vi "HandleObservationSync.vi"(8 "error in (no error)":errorcluster, 11 "S4GUI in":refnum<class "S4GUI.lvclass">) -> (0 "error out":errorcluster, 3 "S4GUI out":refnum<class "S4GUI.lvclass">)   [LabVIEW 2018, in "S4GUI.lvclass"] (continued)
              n1024 = call-dynamic "Read Channel.vi"("error in (no error)"=w2761, "Acquisition in"=w2762) -> ("error out"=w2769:errorcluster, "Channel.lvclass"=w2770:refnum<class "Channel.lvclass">, "Acquisition out"=w2763:refnum<class "Acquisition.lvclass">)  [unwired: 7 in]
              n1025 = call-dynamic "Read State Machine.vi"("error in (no error)"=w2769, "Device in"=w2770) -> ("error out"=w2768:errorcluster, "State Machine.lvclass"=w2766:refnum<class "State Machine.lvclass">, "Device out"=w2772:refnum<class "Channel.lvclass">)  [unwired: 7 in]
              n1026 = call "Next State.vi"("error in (no error)"=w2768, "New_State"=50, "State Machine in"=w2766) -> ("error out"=w2760:errorcluster, "State Machine out"=w2759:refnum<class "State Machine.lvclass">)  [unwired: 7 in]
              n1027 = call-dynamic "Write State Machine.vi"("error in (no error)"=w2760, "State Machine.lvclass"=w2759, "Device in"=w2772) -> ("error out"=w2773:errorcluster, "Device out"=w2771:refnum<class "Channel.lvclass">)  [unwired: 7 in]
              n1028 = call-dynamic "Write Channel.vi"("error in (no error)"=w2773, "Channel.lvclass"=w2771, "Acquisition in"=w2763) -> ("error out"=w2765:errorcluster, "Acquisition out"=w2764:refnum<class "Acquisition.lvclass">)  [unwired: 7 in]
            }
          }
          n1029 = call-dynamic "Write AcquisitionC.vi"("error in (no error)"=w2684, "Acquisition.lvclass"=w2682, "S4ACS_GUI in"=w2683) -> ("error out"=w2678:errorcluster, "S4ACS_GUI out"=w2677:refnum<class "S4GUI.lvclass">)  [unwired: 7 in]
          n1030 = call-dynamic "Read AcquisitionD.vi"("error in (no error)"=w2678, "S4ACS_GUI in"=w2677) -> ("error out"=w2634:errorcluster, "Acquisition.lvclass"=w2636:refnum<class "Acquisition.lvclass">, "S4ACS_GUI out"=w2676:refnum<class "S4GUI.lvclass">)  [unwired: 7 in]
          n1031 = call-dynamic "Read enabled.vi"("error in (no error)"=w2634, "Server in"=w2636) -> ("error out"=w2633:errorcluster, "enabled"=w2629:bool, "Server out"=w2635:refnum<class "Acquisition.lvclass">)  [unwired: 7 in]
          n1032 = call "Read connection.vi"("error in (no error)"=w2633, "Server in"=w2635) -> ("error out"=w2665:errorcluster, "connection"=w2649:bool, "Server out"=w2666:refnum<class "Acquisition.lvclass">)  [unwired: 7 in]
          n1033 = And(x=w2649, y=w2629) -> (x .and. y?=w2651:bool)
          n1034 = case shown="True" w2651 {
            tunnel: w2665 -> [w2734 w2751]
            tunnel: [w2734 w2750] -> w2679
            tunnel: w2666 -> [w2735 w2741]
            tunnel: [w2735 w2739] -> w2675
            tunnel: [w2731 u32 0 ("New_State")] -> w2658
            tunnel: w2629 -> [w2730 _]
            frame False {
              n1035 = Select(t=u32 8, s=w2730, f=u32 0) -> (s? t:f=w2731:u32)
            }
            frame True {
              n1036 = call-dynamic "Read Channel.vi"("error in (no error)"=w2751, "Acquisition in"=w2741) -> ("error out"=w2746:errorcluster, "Channel.lvclass"=w2745:refnum<class "Channel.lvclass">, "Acquisition out"=w2740:refnum<class "Acquisition.lvclass">)  [unwired: 7 in]
              n1037 = call-dynamic "Read State Machine.vi"("error in (no error)"=w2746, "Device in"=w2745) -> ("error out"=w2747:errorcluster, "State Machine.lvclass"=w2749:refnum<class "State Machine.lvclass">, "Device out"=w2743:refnum<class "Channel.lvclass">)  [unwired: 7 in]
              n1038 = call "Next State.vi"("error in (no error)"=w2747, "New_State"=50, "State Machine in"=w2749) -> ("error out"=w2737:errorcluster, "State Machine out"=w2738:refnum<class "State Machine.lvclass">)  [unwired: 7 in]
              n1039 = call-dynamic "Write State Machine.vi"("error in (no error)"=w2737, "State Machine.lvclass"=w2738, "Device in"=w2743) -> ("error out"=w2742:errorcluster, "Device out"=w2744:refnum<class "Channel.lvclass">)  [unwired: 7 in]
              n1040 = call-dynamic "Write Channel.vi"("error in (no error)"=w2742, "Channel.lvclass"=w2744, "Acquisition in"=w2740) -> ("error out"=w2750:errorcluster, "Acquisition out"=w2739:refnum<class "Acquisition.lvclass">)  [unwired: 7 in]
            }
          }
          n1041 = call-dynamic "Write AcquisitionD.vi"("error in (no error)"=w2679, "Acquisition.lvclass"=w2675, "S4ACS_GUI in"=w2676) -> ("error out"=w2674:errorcluster, "S4ACS_GUI out"=w2673:refnum<class "S4GUI.lvclass">)  [unwired: 7 in]
          n1042 = Compound Arithmetic op=ADD(w2661, w2660, w2659, w2658) -> (w2662:u32)
          n1043 = case shown="0, Default" w2662 {
            tunnel: w2657 -> [w2699 _ _ _ _ _ _ _ _ _ _ _ _ _ _ _]
            tunnel: [w2698 u32 1 ("Obs_state") u32 1 ("Obs_state") u32 1 ("Obs_state") u32 1 ("Obs_state") u32 1 ("Obs_state") u32 1 ("Obs_state") u32 1 ("Obs_state") u32 1 ("Obs_state") u32 1 ("Obs_state") u32 1 ("Obs_state") u32 1 ("Obs_state") u32 1 ("Obs_state") u32 1 ("Obs_state") u32 1 ("Obs_state") u32 1 ("Obs_state")] -> w2663
            tunnel: ["" ("Error Msg") "ERROR: Lost channel 1 connection... - HandleObservationSync.vi state 308" ("Error Msg") "ERROR: Lost channel 2 connection...- HandleObservationSync.vi state 308" ("Error Msg") "ERROR: Lost channels 1 and 2 connection...- HandleObservationSync.vi state 308" ("Error Msg") "ERROR: Lost channel 3 connection...- HandleObservationSync.vi state 308" ("Error Msg") "ERROR: Lost channels 1 and  3 connection...- HandleObservationSync.vi state 308" ("Error Msg") "ERROR:  Lost channels 2 and  3 connection...- HandleObservationSync.vi state 308" ("Error Msg") "ERROR:  Lost channels 1, 2 and  3 connection...- HandleObservationSync.vi state 308" ("Error Msg") "ERROR: Lost channel 4 connection...- HandleObservationSync.vi state 308" ("Error Msg") "ERROR:  Lost channels 1 and 4 connection...- HandleObservationSync.vi state 308" ("Error Msg") "ERROR:  Lost channels 2 and 4 connection...- HandleObservationSync.vi state 308" ("Error Msg") "ERROR: Lost channels 1, 2 and 4 connection...- HandleObservationSync.vi state 308" ("Error Msg") "ERROR: Lost channels 3 and 4 connection...- HandleObservationSync.vi state 308" ("Error Msg") "ERROR: Lost channels 1, 3 and 4 connection...- HandleObservationSync.vi state 308" ("Error Msg") "ERROR: Lost channels 2, 3 and 4 connection...- HandleObservationSync.vi state 308" ("Error Msg") "ERROR: Lost channels 1, 2, 3 and 4 connection...- HandleObservationSync.vi state 308" ("Error Msg")] -> w2664
            frame 0, Default {
              n1044 = Tick Count (ms)() -> (millisecond timer value=w2696:u32)
              n1045 = Increment(x=w2699) -> (x+1=w2698:u32)
              n1046 = local write "time1"(w2696) -> ()
            }
            frame 1 {
            }
            frame 2 {
            }
            frame 3 {
            }
            frame 4 {
            }
            frame 5 {
            }
            frame 6 {
            }
            frame 7 {
            }
            frame 8 {
            }
            frame 9 {
            }
            frame 10 {
            }
            frame 11 {
            }
            frame 12 {
            }
            frame 13 {
            }
            frame 14 {
            }
            frame 15 {
            }
          }
          n1047 = Bundle By Name(cluster=w2673, "Obs_state"=w2663, "Error Msg"=w2664) -> (w2690:refnum<class "S4GUI.lvclass">)
        }
        frame 309 {
          # "Se wait_expose=T, não envia\no EXPOSE do estado 310\n(1o EXPOSE já foi enviado).\n\nNeste caso, vai para:\n* 310 se houver mais \n   de 1 posição da lamina ou para \n* 327 se houver apenas 1 posição\n   da lâmina"
          # "T: mode EXPOSE\nF: mode FIRE"
          n1048 = Unbundle By Name(w2824) -> ("seqAtual"=w2823:u32)
          n1049 = call-dynamic "Read AcquisitionA.vi"("error in (no error)"=w2884, "S4ACS_GUI in"=w2824) -> ("error out"=w2864:errorcluster, "Acquisition.lvclass"=w2865:refnum<class "Acquisition.lvclass">, "S4ACS_GUI out"=w2886:refnum<class "S4GUI.lvclass">)  [unwired: 7 in]
          n1050 = call "Read connection.vi"("error in (no error)"=w2864, "Server in"=w2865) -> ("error out"=w2866:errorcluster, "connection"=w2868:bool, "Server out"=w2867:refnum<class "Acquisition.lvclass">)  [unwired: 7 in]
          n1051 = case shown="True" w2868 {
            tunnel: [w3037 w3061] -> w2887
            tunnel: [w3036 w3060] -> w2885
            tunnel: w2867 -> [w3037 w3053]
            tunnel: w2866 -> [w3036 w3052]
            tunnel: [TRUE w3051] -> w2847
            tunnel: [FALSE w3045] -> w2843
            tunnel: [TRUE w3039] -> w2828
            tunnel: w2823 -> [_ w3038]
            frame False {
            }
            frame True {
              n1052 = call-dynamic "Read Channel.vi"("error in (no error)"=w3052, "Acquisition in"=w3053) -> ("error out"=w3042:errorcluster, "Channel.lvclass"=w3044:refnum<class "Channel.lvclass">, "Acquisition out"=w3062:refnum<class "Acquisition.lvclass">)  [unwired: 7 in]
              n1053 = call-dynamic "Read SequesDone.vi"("error in (no error)"=w3042, "Channel in"=w3044) -> ("error out"=w3041:errorcluster, "SequesDoneRaw"=w3040:u32, "Channel out"=w3043:refnum<class "Channel.lvclass">)  [unwired: 6 in, 1 out]
              n1054 = Equal?(x=w3040, y=w3038) -> (x = y?=w3039:bool)
              n1055 = call-dynamic "Read wait_expose.vi"("error in (no error)"=w3041, "Channel in"=w3043) -> ("error out"=w3046:errorcluster, "wait_expose"=w3045:bool, "Channel out"=w3047:refnum<class "Channel.lvclass">)  [unwired: 7 in]
              n1056 = call-dynamic "Read State Machine.vi"("error in (no error)"=w3046, "Device in"=w3047) -> ("error out"=w3054:errorcluster, "State Machine.lvclass"=w3056:refnum<class "State Machine.lvclass">, "Device out"=w3058:refnum<class "Channel.lvclass">)  [unwired: 7 in]
              n1057 = call-dynamic "Read State.vi"("error in (no error)"=w3054, "State Machine in"=w3056) -> ("error out"=w3048:errorcluster, "State"=w3050:i32, "State Machine out"=w3055:refnum<class "State Machine.lvclass">)  [unwired: 7 in]
              n1058 = Greater?(x=w3050, y=53) -> (0:w3051:bool)
              n1059 = call-dynamic "Write State Machine.vi"("error in (no error)"=w3048, "State Machine.lvclass"=w3055, "Device in"=w3058) -> ("error out"=w3057:errorcluster, "Device out"=w3059:refnum<class "Channel.lvclass">)  [unwired: 7 in]
              n1060 = call-dynamic "Write Channel.vi"("error in (no error)"=w3057, "Channel.lvclass"=w3059, "Acquisition in"=w3062) -> ("error out"=w3060:errorcluster, "Acquisition out"=w3061:refnum<class "Acquisition.lvclass">)  [unwired: 7 in]
            }
          }
          n1061 = call-dynamic "Write AcquisitionA.vi"("error in (no error)"=w2885, "Acquisition.lvclass"=w2887, "S4ACS_GUI in"=w2886) -> ("error out"=w2881:errorcluster, "S4ACS_GUI out"=w2882:refnum<class "S4GUI.lvclass">)  [unwired: 7 in]
          n1062 = call "Read AcquisitionB.vi"("error in (no error)"=w2881, "S4ACS_GUI in"=w2882) -> ("error out"=w2861:errorcluster, "Acquisition.lvclass"=w2863:refnum<class "Acquisition.lvclass">, "S4ACS_GUI out"=w2879:refnum<class "S4GUI.lvclass">)  [unwired: 7 in]
          n1063 = call "Read connection.vi"("error in (no error)"=w2861, "Server in"=w2863) -> ("error out"=w2860:errorcluster, "connection"=w2859:bool, "Server out"=w2862:refnum<class "Acquisition.lvclass">)  [unwired: 7 in]
          n1064 = case shown="True" w2859 {
            tunnel: w2862 -> [w3007 w3032]
            tunnel: w2860 -> [w3006 w3031]
            tunnel: [w3007 w3029] -> w2880
            tunnel: [w3006 w3028] -> w2878
            tunnel: [TRUE w3019] -> w2846
            tunnel: [FALSE ("expose") w3015] -> w2842
            tunnel: [TRUE w3009] -> w2830
            tunnel: w2823 -> [_ w3008]
            frame False {
            }
            frame True {
              n1065 = call-dynamic "Read Channel.vi"("error in (no error)"=w3031, "Acquisition in"=w3032) -> ("error out"=w3011:errorcluster, "Channel.lvclass"=w3014:refnum<class "Channel.lvclass">, "Acquisition out"=w3030:refnum<class "Acquisition.lvclass">)  [unwired: 7 in]
              n1066 = call-dynamic "Read SequesDone.vi"("error in (no error)"=w3011, "Channel in"=w3014) -> ("error out"=w3010:errorcluster, "SequesDoneRaw"=w3012:u32, "Channel out"=w3013:refnum<class "Channel.lvclass">)  [unwired: 6 in, 1 out]
              n1067 = Equal?(x=w3012, y=w3008) -> (x = y?=w3009:bool)
              n1068 = call-dynamic "Read wait_expose.vi"("error in (no error)"=w3010, "Channel in"=w3013) -> ("error out"=w3016:errorcluster, "wait_expose"=w3015:bool, "Channel out"=w3017:refnum<class "Channel.lvclass">)  [unwired: 7 in]
              n1069 = call-dynamic "Read State Machine.vi"("error in (no error)"=w3016, "Device in"=w3017) -> ("error out"=w3022:errorcluster, "State Machine.lvclass"=w3024:refnum<class "State Machine.lvclass">, "Device out"=w3026:refnum<class "Channel.lvclass">)  [unwired: 7 in]
              n1070 = call-dynamic "Read State.vi"("error in (no error)"=w3022, "State Machine in"=w3024) -> ("error out"=w3021:errorcluster, "State"=w3018:i32, "State Machine out"=w3023:refnum<class "State Machine.lvclass">)  [unwired: 7 in]
              n1071 = Greater?(x=w3018, y=53) -> (0:w3019:bool)
              n1072 = call-dynamic "Write State Machine.vi"("error in (no error)"=w3021, "State Machine.lvclass"=w3023, "Device in"=w3026) -> ("error out"=w3025:errorcluster, "Device out"=w3027:refnum<class "Channel.lvclass">)  [unwired: 7 in]
              n1073 = call-dynamic "Write Channel.vi"("error in (no error)"=w3025, "Channel.lvclass"=w3027, "Acquisition in"=w3030) -> ("error out"=w3028:errorcluster, "Acquisition out"=w3029:refnum<class "Acquisition.lvclass">)  [unwired: 7 in]
            }
          }
          n1074 = call "Write AcquisitionB.vi"("error in (no error)"=w2878, "Acquisition.lvclass"=w2880, "S4ACS_GUI in"=w2879) -> ("error out"=w2874:errorcluster, "S4ACS_GUI out"=w2873:refnum<class "S4GUI.lvclass">)  [unwired: 7 in]
          n1075 = call-dynamic "Read AcquisitionC.vi"("error in (no error)"=w2874, "S4ACS_GUI in"=w2873) -> ("error out"=w2856:errorcluster, "Acquisition.lvclass"=w2858:refnum<class "Acquisition.lvclass">, "S4ACS_GUI out"=w2876:refnum<class "S4GUI.lvclass">)  [unwired: 7 in]
          n1076 = call "Read connection.vi"("error in (no error)"=w2856, "Server in"=w2858) -> ("error out"=w2855:errorcluster, "connection"=w2854:bool, "Server out"=w2857:refnum<class "Acquisition.lvclass">)  [unwired: 7 in]
          n1077 = case shown="True" w2854 {
            tunnel: [w2976 w2997] -> w2877
            tunnel: [w2977 w2996] -> w2875
            tunnel: w2857 -> [w2977 w2992]
            tunnel: w2855 -> [w2976 w2991]
            tunnel: [TRUE w2988] -> w2845
            tunnel: [FALSE ("expose") w2985] -> w2841
            tunnel: [TRUE w2979] -> w2829
            tunnel: w2823 -> [_ w2978]
            frame False {
            }
            frame True {
              n1078 = call-dynamic "Read Channel.vi"("error in (no error)"=w2991, "Acquisition in"=w2992) -> ("error out"=w2984:errorcluster, "Channel.lvclass"=w2983:refnum<class "Channel.lvclass">, "Acquisition out"=w2995:refnum<class "Acquisition.lvclass">)  [unwired: 7 in]
              n1079 = call-dynamic "Read SequesDone.vi"("error in (no error)"=w2984, "Channel in"=w2983) -> ("error out"=w2980:errorcluster, "SequesDoneRaw"=w2981:u32, "Channel out"=w2982:refnum<class "Channel.lvclass">)  [unwired: 6 in, 1 out]
              n1080 = Equal?(x=w2981, y=w2978) -> (x = y?=w2979:bool)
              n1081 = call-dynamic "Read wait_expose.vi"("error in (no error)"=w2980, "Channel in"=w2982) -> ("error out"=w2986:errorcluster, "wait_expose"=w2985:bool, "Channel out"=w2987:refnum<class "Channel.lvclass">)  [unwired: 7 in]
              n1082 = call-dynamic "Read State Machine.vi"("error in (no error)"=w2986, "Device in"=w2987) -> ("error out"=w2993:errorcluster, "State Machine.lvclass"=w3001:refnum<class "State Machine.lvclass">, "Device out"=w2999:refnum<class "Channel.lvclass">)  [unwired: 7 in]
              n1083 = call-dynamic "Read State.vi"("error in (no error)"=w2993, "State Machine in"=w3001) -> ("error out"=w2994:errorcluster, "State"=w2989:i32, "State Machine out"=w3002:refnum<class "State Machine.lvclass">)  [unwired: 7 in]
              n1084 = Greater?(x=w2989, y=53) -> (0:w2988:bool)
              n1085 = call-dynamic "Write State Machine.vi"("error in (no error)"=w2994, "State Machine.lvclass"=w3002, "Device in"=w2999) -> ("error out"=w3000:errorcluster, "Device out"=w2998:refnum<class "Channel.lvclass">)  [unwired: 7 in]
              n1086 = call-dynamic "Write Channel.vi"("error in (no error)"=w3000, "Channel.lvclass"=w2998, "Acquisition in"=w2995) -> ("error out"=w2997:errorcluster, "Acquisition out"=w2996:refnum<class "Acquisition.lvclass">)  [unwired: 7 in]
            }
          }
          n1087 = call-dynamic "Write AcquisitionC.vi"("error in (no error)"=w2877, "Acquisition.lvclass"=w2875, "S4ACS_GUI in"=w2876) -> ("error out"=w2853:errorcluster, "S4ACS_GUI out"=w2869:refnum<class "S4GUI.lvclass">)  [unwired: 7 in]
          n1088 = call-dynamic "Read AcquisitionD.vi"("error in (no error)"=w2853, "S4ACS_GUI in"=w2869) -> ("error out"=w2849:errorcluster, "Acquisition.lvclass"=w2852:refnum<class "Acquisition.lvclass">, "S4ACS_GUI out"=w2871:refnum<class "S4GUI.lvclass">)  [unwired: 7 in]
          n1089 = call "Read connection.vi"("error in (no error)"=w2849, "Server in"=w2852) -> ("error out"=w2850:errorcluster, "connection"=w2848:bool, "Server out"=w2851:refnum<class "Acquisition.lvclass">)  [unwired: 7 in]
          n1090 = case shown="True" w2848 {
            tunnel: [w2947 w2971] -> w2872
            tunnel: [w2946 w2970] -> w2870
            tunnel: [TRUE w2959] -> w2844
            tunnel: w2851 -> [w2947 w2962]
            tunnel: w2850 -> [w2946 w2961]
            tunnel: [FALSE ("expose") w2955] -> w2840
            tunnel: [TRUE w2949] -> w2831
            tunnel: w2823 -> [_ w2948]
            frame False {
            }
            frame True {
              n1091 = call-dynamic "Read Channel.vi"("error in (no error)"=w2961, "Acquisition in"=w2962) -> ("error out"=w2953:errorcluster, "Channel.lvclass"=w2954:refnum<class "Channel.lvclass">, "Acquisition out"=w2972:refnum<class "Acquisition.lvclass">)  [unwired: 7 in]
              n1092 = call-dynamic "Read SequesDone.vi"("error in (no error)"=w2953, "Channel in"=w2954) -> ("error out"=w2951:errorcluster, "SequesDoneRaw"=w2952:u32, "Channel out"=w2950:refnum<class "Channel.lvclass">)  [unwired: 6 in, 1 out]
              n1093 = Equal?(x=w2952, y=w2948) -> (x = y?=w2949:bool)
              n1094 = call-dynamic "Read wait_expose.vi"("error in (no error)"=w2951, "Channel in"=w2950) -> ("error out"=w2956:errorcluster, "wait_expose"=w2955:bool, "Channel out"=w2957:refnum<class "Channel.lvclass">)  [unwired: 7 in]
              n1095 = call-dynamic "Read State Machine.vi"("error in (no error)"=w2956, "Device in"=w2957) -> ("error out"=w2964:errorcluster, "State Machine.lvclass"=w2966:refnum<class "State Machine.lvclass">, "Device out"=w2968:refnum<class "Channel.lvclass">)  [unwired: 7 in]
              n1096 = call-dynamic "Read State.vi"("error in (no error)"=w2964, "State Machine in"=w2966) -> ("error out"=w2963:errorcluster, "State"=w2958:i32, "State Machine out"=w2965:refnum<class "State Machine.lvclass">)  [unwired: 7 in]
              n1097 = Greater?(x=w2958, y=53) -> (0:w2959:bool)
              n1098 = call-dynamic "Write State Machine.vi"("error in (no error)"=w2963, "State Machine.lvclass"=w2965, "Device in"=w2968) -> ("error out"=w2967:errorcluster, "Device out"=w2969:refnum<class "Channel.lvclass">)  [unwired: 7 in]
              n1099 = call-dynamic "Write Channel.vi"("error in (no error)"=w2967, "Channel.lvclass"=w2969, "Acquisition in"=w2972) -> ("error out"=w2970:errorcluster, "Acquisition out"=w2971:refnum<class "Acquisition.lvclass">)  [unwired: 7 in]
            }
          }
          n1100 = call-dynamic "Write AcquisitionD.vi"("error in (no error)"=w2870, "Acquisition.lvclass"=w2872, "S4ACS_GUI in"=w2871) -> ("error out"=w2822:errorcluster, "S4ACS_GUI out"=w2820:refnum<class "S4GUI.lvclass">)  [unwired: 7 in]
          n1101 = Compound Arithmetic op=OR(w2843, w2842, w2841, w2840) -> (w2833:bool)
          n1102 = Compound Arithmetic op=AND(w2828, w2830, w2829, w2831) -> (w2826:bool)
          n1103 = Compound Arithmetic op=AND(w2847, w2846, w2845, w2844) -> (w2827:bool)
          n1104 = disable-structure shown="Enabled" {
            disable-tunnel: w2827 -> [w2890 w2891]
            disable-tunnel: w2826 -> [w2889 _]
            disable-tunnel: [w2888 w2891] -> w2825
            frame Disabled {
              # "Espera todos os canais chegarem ao estado ACTIVE\n(estados 54 e 55 de Channel:Run.vi)\n   OU\nTodos os canais incrementarem o Seqs_done. (OV 20240821)"
              n1105 = Or(x=w2890, y=w2889) -> (x .or. y?=w2888:bool)
            }
            frame Enabled {
              # "OV20241108:\nEspera APENAS o ACTIVE."
            }
          }
          n1106 = call-dynamic "VerifErrors.vi"("error in (no error)"=w2822, "S4GUI in"=w2820) -> ("error out"=w2821:errorcluster, "Error value"=w2818:u32, "S4GUI out"=w2819:refnum<class "S4GUI.lvclass">)  [unwired: 7 in]
          n1107 = call-dynamic "VerifWavePlate.vi"("error in (no error)"=w2821, "S4GUI in"=w2819) -> ("error out"=w2837:errorcluster, "One Position"=w2839:bool, "S4GUI out"=w2838:refnum<class "S4GUI.lvclass">)  [unwired: 7 in]
          n1108 = case shown="False" w2839 {
            tunnel: w2838 -> [w2924 w2941]
            tunnel: [u32 312 ("t") u32 328 ("t")] -> w2835
            tunnel: [w2924 w2927] -> w2834
            tunnel: w2837 -> [w2922 w2926]
            tunnel: [w2922 w2925] -> w2836
            frame False {
            }
            frame True {
              # "Recarrega SEQ, antes de desviar\n para tratamento de fotometria."
              n1109 = call "Read Instrument.lvclass.vi"("error in (no error)"=w2926, "S4ACS_GUI in"=w2941) -> ("error out"=w2936:errorcluster, "Instrument.lvclass"=w2940:refnum<class "Instrument.lvclass">, "S4ACS_GUI out"=w2939:refnum<class "S4GUI.lvclass">)  [unwired: 7 in]
              n1110 = call "Read WPROT.vi"("error in (no error)"=w2936, "Instrument in"=w2940) -> ("error out"=w2929:errorcluster, "Opt_Selector.lvclass"=w2932:refnum<class "Opt_Selector.lvclass">, "Instrument out"=w2937:refnum<class "Instrument.lvclass">)  [unwired: 7 in]
              n1111 = call-dynamic "Read sequencia_ant.vi"("error in (no error)"=w2929, "Opt_Selector in"=w2932) -> ("error out"=w2934:errorcluster, "sequencia_ant"=w2933:u16, "Opt_Selector out"=w2931:refnum<class "Opt_Selector.lvclass">)  [unwired: 7 in]
              n1112 = call-dynamic "Write sequencia.vi"("error in (no error)"=w2934, "sequencia"=w2933, "Opt_Selector in"=w2931) -> ("error out"=w2928:errorcluster, "Opt_Selector out"=w2930:refnum<class "Opt_Selector.lvclass">)  [unwired: 7 in]
              n1113 = call "Write WPROT.vi"("error in (no error)"=w2928, "Opt_Selector.lvclass"=w2930, "Instrument in"=w2937) -> ("error out"=w2935:errorcluster, "Instrument out"=w2938:refnum<class "Instrument.lvclass">)  [unwired: 7 in]
              n1114 = call "Write Instrument.lvclass.vi"("error in (no error)"=w2935, "Instrument.lvclass"=w2938, "S4ACS_GUI in"=w2939) -> ("error out"=w2925:errorcluster, "S4ACS_GUI out"=w2927:refnum<class "S4GUI.lvclass">)  [unwired: 7 in]
            }
          }
          n1115 = case shown="False" w2825 {
            tunnel: w2834 -> [w2894 w2921]
            tunnel: [w2900 w2920] -> w2832
            tunnel: w2835 -> [_ w2918]
            tunnel: w2818 -> [w2892 _]
            frame False {
              # "Aguardando iniciar exposição por 5s"
              n1116 = Tick Count (ms)() -> (millisecond timer value=w2899:u32)
              n1117 = local read "time1"() -> (w2893:u32)
              n1118 = Subtract(x=w2899, y=w2893) -> (x-y=w2896:u32)
              n1119 = To Double Precision Float(number=w2896) -> (double precision float=w2898:dbl)
              n1120 = Less?(x=5000.0 ("y"), y=w2898) -> (x < y?=w2897:bool)
              n1121 = case shown="False" w2897 {
                tunnel: w2894 -> [w2902 w2916]
                tunnel: [w2901 w2915] -> w2900
                tunnel: w2892 -> [w2903 _]
                frame False {
                  n1122 = case shown="1..15" w2903 {
                    selector: w2903 -> [_ w2911]
                    tunnel: [w2904 w2906] -> w2901
                    tunnel: w2902 -> [w2904 w2912]
                    frame 0, Default {
                    }
                    frame 1..15 {
                      n1123 = Number To Decimal String(number=w2911) -> (decimal integer string=w2908:string)  [unwired: 1 in]
                      n1124 = Concatenate Strings("CHANNEL ERROR <", w2908, ">: Error flag TRUE - see ACS panel.  HandleObservationSync.vi - state 309.") -> (w2910:string)
                      n1125 = Bundle By Name(cluster=w2912, "Obs_state"=u32 1, "Error Msg"=w2910) -> (w2906:refnum<class "S4GUI.lvclass">)
                    }
                  }
                }
                frame True {
                  n1126 = Bundle By Name(cluster=w2916, "Obs_state"=u32 1, "Error Msg"="ERROR: Acquisition Timeout. HandleObservationSync.vi - state 309.") -> (w2915:refnum<class "S4GUI.lvclass">)
                }
              }
            }
            frame True {
              # "Iniciou aquisição..."
              n1127 = Tick Count (ms)() -> (millisecond timer value=→"time308":u32)
              n1128 = Tick Count (ms)() -> (millisecond timer value=w2919:u32)
              n1129 = Bundle By Name(cluster=w2921, "Obs_state"=w2918) -> (w2920:refnum<class "S4GUI.lvclass">)
              n1130 = local write "time307"(w2919) -> ()
              n1131 = local write "time1"(w2919) -> ()
            }
          }
          n1132 = Bundle By Name(cluster=w2832, "mode EXPOSE"=w2833) -> (w2883:refnum<class "S4GUI.lvclass">)
        }
        frame 312 {
          # "Verifcando avanço de SEQUENCIA:"
          # "T=canais receberam STOP"
          # "T= Todos os canais ativos na mesma sequencia;\nF= Canais com sequencia diferente"
          # "Todos os SEQ_DONE \nsão iguais a SeqAtual?\nSe sim, avança lâmina."
          # "Exemplo:\nSET #CYCLES 3\nSET #SEQ 4\ntotal de sequencias: 3 x 4 = 12\n\nseq.        CYCLES_DONE           SEQS_DONE\n1a.                     0                                 0\n2a.                     0                                 1 \n3a.                     0                                 2 \n4a.                     0                                 3 \n                          1                                 4\n5a.                     1                                 0 \n6a.                     1                                 1 \n7a.                     1                                 2 \n8a.                     1                                 3 \n                          2                                 4\n9a.                     2                                 0 \n10a.                   2                                 1 \n11a.                   2                                 2 \n12a.                   2                                 3 \n\nfim                    3                                 4"
          n1133 = Unbundle By Name(w3088) -> ("seqAtual"=w3085:u32)
          n1134 = call-dynamic "Read AcquisitionA.vi"("error in (no error)"=w3122, "S4ACS_GUI in"=w3088) -> ("error out"=w3103:errorcluster, "Acquisition.lvclass"=w3104:refnum<class "Acquisition.lvclass">, "S4ACS_GUI out"=w3124:refnum<class "S4GUI.lvclass">)  [unwired: 7 in]
          n1135 = call-dynamic "Read enabled.vi"("error in (no error)"=w3103, "Server in"=w3104) -> ("error out"=w3102:errorcluster, "enabled"=w3077:bool, "Server out"=w3101:refnum<class "Acquisition.lvclass">)  [unwired: 7 in]
          n1136 = case shown="True" w3077 {
            tunnel: w3102 -> [w3273 w3289]
            tunnel: [w3274 w3287] -> w3125
            tunnel: [w3273 w3286] -> w3123
            tunnel: [u32 0 ("SequesDone") w3275] -> w3082
            tunnel: w3101 -> [w3274 w3285]
            tunnel: w3085 -> [_ w3284]
            tunnel: [TRUE w3283] -> w3087
            tunnel: [FALSE ("stopping") w3276] -> w3070
            frame False {
            }
            frame True {
              # "SEQS_DONE = 0,1,2,...,n,0,1,..."
              n1137 = call-dynamic "Read Channel.vi"("error in (no error)"=w3289, "Acquisition in"=w3285) -> ("error out"=w3281:errorcluster, "Channel.lvclass"=w3282:refnum<class "Channel.lvclass">, "Acquisition out"=w3288:refnum<class "Acquisition.lvclass">)  [unwired: 7 in]
              n1138 = call-dynamic "Read SequesDone.vi"("error in (no error)"=w3281, "Channel in"=w3282) -> ("error out"=w3279:errorcluster, "SequesDoneRaw"=w3275:u32, "Channel out"=w3280:refnum<class "Channel.lvclass">)  [unwired: 6 in, 1 out]
              n1139 = Equal?(x=w3275, y=w3284) -> (x = y?=w3283:bool)
              n1140 = call-dynamic "Read stopping.vi"("error in (no error)"=w3279, "Channel in"=w3280) -> ("error out"=w3278:errorcluster, "stopping"=w3276:bool, "Channel out"=w3277:refnum<class "Channel.lvclass">)  [unwired: 7 in]
              n1141 = call-dynamic "Write Channel.vi"("error in (no error)"=w3278, "Channel.lvclass"=w3277, "Acquisition in"=w3288) -> ("error out"=w3286:errorcluster, "Acquisition out"=w3287:refnum<class "Acquisition.lvclass">)  [unwired: 7 in]
            }
          }
          n1142 = call-dynamic "Write AcquisitionA.vi"("error in (no error)"=w3123, "Acquisition.lvclass"=w3125, "S4ACS_GUI in"=w3124) -> ("error out"=w3120:errorcluster, "S4ACS_GUI out"=w3119:refnum<class "S4GUI.lvclass">)  [unwired: 7 in]
          n1143 = call "Read AcquisitionB.vi"("error in (no error)"=w3120, "S4ACS_GUI in"=w3119) -> ("error out"=w3097:errorcluster, "Acquisition.lvclass"=w3100:refnum<class "Acquisition.lvclass">, "S4ACS_GUI out"=w3121:refnum<class "S4GUI.lvclass">)  [unwired: 7 in]
          n1144 = call-dynamic "Read enabled.vi"("error in (no error)"=w3097, "Server in"=w3100) -> ("error out"=w3098:errorcluster, "enabled"=w3076:bool, "Server out"=w3099:refnum<class "Acquisition.lvclass">)  [unwired: 7 in]
          n1145 = case shown="True" w3076 {
            tunnel: w3098 -> [w3253 w3269]
            tunnel: w3099 -> [w3254 w3268]
            tunnel: [u32 0 ("SequesDone") w3255] -> w3079
            tunnel: [w3253 w3267] -> w3118
            tunnel: [w3254 w3266] -> w3117
            tunnel: w3085 -> [_ w3263]
            tunnel: [TRUE w3262] -> w3086
            tunnel: [FALSE ("stopping") w3256] -> w3069
            frame False {
            }
            frame True {
              n1146 = call-dynamic "Read Channel.vi"("error in (no error)"=w3269, "Acquisition in"=w3268) -> ("error out"=w3260:errorcluster, "Channel.lvclass"=w3261:refnum<class "Channel.lvclass">, "Acquisition out"=w3264:refnum<class "Acquisition.lvclass">)  [unwired: 7 in]
              n1147 = call-dynamic "Read SequesDone.vi"("error in (no error)"=w3260, "Channel in"=w3261) -> ("error out"=w3258:errorcluster, "SequesDoneRaw"=w3255:u32, "Channel out"=w3265:refnum<class "Channel.lvclass">)  [unwired: 6 in, 1 out]
              n1148 = Equal?(x=w3255, y=w3263) -> (x = y?=w3262:bool)
              n1149 = call-dynamic "Read stopping.vi"("error in (no error)"=w3258, "Channel in"=w3265) -> ("error out"=w3257:errorcluster, "stopping"=w3256:bool, "Channel out"=w3259:refnum<class "Channel.lvclass">)  [unwired: 7 in]
              n1150 = call-dynamic "Write Channel.vi"("error in (no error)"=w3257, "Channel.lvclass"=w3259, "Acquisition in"=w3264) -> ("error out"=w3267:errorcluster, "Acquisition out"=w3266:refnum<class "Acquisition.lvclass">)  [unwired: 7 in]
            }
          }
          n1151 = call "Write AcquisitionB.vi"("error in (no error)"=w3118, "Acquisition.lvclass"=w3117, "S4ACS_GUI in"=w3121) -> ("error out"=w3110:errorcluster, "S4ACS_GUI out"=w3109:refnum<class "S4GUI.lvclass">)  [unwired: 7 in]
          n1152 = call-dynamic "Read AcquisitionC.vi"("error in (no error)"=w3110, "S4ACS_GUI in"=w3109) -> ("error out"=w3094:errorcluster, "Acquisition.lvclass"=w3096:refnum<class "Acquisition.lvclass">, "S4ACS_GUI out"=w3112:refnum<class "S4GUI.lvclass">)  [unwired: 7 in]
          n1153 = call-dynamic "Read enabled.vi"("error in (no error)"=w3094, "Server in"=w3096) -> ("error out"=w3093:errorcluster, "enabled"=w3075:bool, "Server out"=w3095:refnum<class "Acquisition.lvclass">)  [unwired: 7 in]
          n1154 = case shown="True" w3075 {
            tunnel: [w3233 w3249] -> w3113
            tunnel: [w3234 w3248] -> w3111
            tunnel: w3093 -> [w3233 w3245]
            tunnel: w3095 -> [w3234 w3246]
            tunnel: [u32 0 ("SequesDone") w3235] -> w3078
            tunnel: w3085 -> [_ w3244]
            tunnel: [TRUE w3243] -> w3084
            tunnel: [FALSE ("stopping") w3236] -> w3068
            frame False {
            }
            frame True {
              n1155 = call-dynamic "Read Channel.vi"("error in (no error)"=w3245, "Acquisition in"=w3246) -> ("error out"=w3240:errorcluster, "Channel.lvclass"=w3241:refnum<class "Channel.lvclass">, "Acquisition out"=w3247:refnum<class "Acquisition.lvclass">)  [unwired: 7 in]
              n1156 = call-dynamic "Read SequesDone.vi"("error in (no error)"=w3240, "Channel in"=w3241) -> ("error out"=w3238:errorcluster, "SequesDoneRaw"=w3235:u32, "Channel out"=w3242:refnum<class "Channel.lvclass">)  [unwired: 6 in, 1 out]
              n1157 = Equal?(x=w3235, y=w3244) -> (x = y?=w3243:bool)
              n1158 = call-dynamic "Read stopping.vi"("error in (no error)"=w3238, "Channel in"=w3242) -> ("error out"=w3237:errorcluster, "stopping"=w3236:bool, "Channel out"=w3239:refnum<class "Channel.lvclass">)  [unwired: 7 in]
              n1159 = call-dynamic "Write Channel.vi"("error in (no error)"=w3237, "Channel.lvclass"=w3239, "Acquisition in"=w3247) -> ("error out"=w3249:errorcluster, "Acquisition out"=w3248:refnum<class "Acquisition.lvclass">)  [unwired: 7 in]
            }
          }
          n1160 = call-dynamic "Write AcquisitionC.vi"("error in (no error)"=w3113, "Acquisition.lvclass"=w3111, "S4ACS_GUI in"=w3112) -> ("error out"=w3107:errorcluster, "S4ACS_GUI out"=w3108:refnum<class "S4GUI.lvclass">)  [unwired: 7 in]
          n1161 = call-dynamic "Read AcquisitionD.vi"("error in (no error)"=w3107, "S4ACS_GUI in"=w3108) -> ("error out"=w3090:errorcluster, "Acquisition.lvclass"=w3092:refnum<class "Acquisition.lvclass">, "S4ACS_GUI out"=w3114:refnum<class "S4GUI.lvclass">)  [unwired: 7 in]
          n1162 = call-dynamic "Read enabled.vi"("error in (no error)"=w3090, "Server in"=w3092) -> ("error out"=w3089:errorcluster, "enabled"=w3074:bool, "Server out"=w3091:refnum<class "Acquisition.lvclass">)  [unwired: 7 in]
          n1163 = Build Array(w3077, w3076, w3075, w3074) -> (w3073:bool[])
          n1164 = case shown="True" w3074 {
            tunnel: [w3214 w3229] -> w3116
            tunnel: [w3213 w3228] -> w3115
            tunnel: w3091 -> [w3214 w3227]
            tunnel: w3089 -> [w3213 w3226]
            tunnel: [u32 0 ("SequesDone") w3215] -> w3081
            tunnel: w3085 -> [_ w3224]
            tunnel: [TRUE w3223] -> w3083
            tunnel: [FALSE ("stopping") w3216] -> w3067
            frame False {
            }
            frame True {
              n1165 = call-dynamic "Read Channel.vi"("error in (no error)"=w3226, "Acquisition in"=w3227) -> ("error out"=w3220:errorcluster, "Channel.lvclass"=w3221:refnum<class "Channel.lvclass">, "Acquisition out"=w3225:refnum<class "Acquisition.lvclass">)  [unwired: 7 in]
              n1166 = call-dynamic "Read SequesDone.vi"("error in (no error)"=w3220, "Channel in"=w3221) -> ("error out"=w3218:errorcluster, "SequesDoneRaw"=w3215:u32, "Channel out"=w3222:refnum<class "Channel.lvclass">)  [unwired: 6 in, 1 out]
              n1167 = Equal?(x=w3215, y=w3224) -> (x = y?=w3223:bool)
              n1168 = call-dynamic "Read stopping.vi"("error in (no error)"=w3218, "Channel in"=w3222) -> ("error out"=w3217:errorcluster, "stopping"=w3216:bool, "Channel out"=w3219:refnum<class "Channel.lvclass">)  [unwired: 7 in]
              n1169 = call-dynamic "Write Channel.vi"("error in (no error)"=w3217, "Channel.lvclass"=w3219, "Acquisition in"=w3225) -> ("error out"=w3228:errorcluster, "Acquisition out"=w3229:refnum<class "Acquisition.lvclass">)  [unwired: 7 in]
            }
          }
          n1170 = Boolean Array To Number(Boolean array=w3073) -> (number=w3071:u32)
          n1171 = Compound Arithmetic op=AND(w3087, w3086, w3084, w3083) -> (w3072:bool)
          n1172 = Compound Arithmetic op=OR(w3070, w3069, w3068, w3067) -> (w3066:bool)
          n1173 = case shown="11" w3071 {
            tunnel: w3082 -> [w3133 _ w3145 _ w3154 _ w3160 w3166 _ w3172 w3175 _]
            tunnel: w3081 -> [w3132 w3136 w3141 w3148 w3149 w3157 w3159 _ _ _ _ _]
            tunnel: w3079 -> [w3131 w3134 _ _ w3153 w3155 _ w3165 w3169 _ w3174 _]
            tunnel: w3078 -> [w3130 w3135 w3140 w3146 _ _ _ w3164 w3168 w3171 _ _]
            tunnel: [w3126 w3137 w3142 w3147 w3150 w3156 w3158 w3161 w3167 w3170 w3173 TRUE] -> _
            frame 15 {
              # "A,B,C,D ativos"
              n1174 = Equal?(x=w3133, y=w3131) -> (x = y?=w3129:bool)
              n1175 = Equal?(x=w3130, y=w3132) -> (x = y?=w3127:bool)
              n1176 = Equal?(x=w3131, y=w3130) -> (x = y?=w3128:bool)
              n1177 = Compound Arithmetic op=AND(w3129, w3128, w3127) -> (w3126:bool)
            }
            frame 14 {
              # "B,C e,D ativos"
              n1178 = Equal?(x=w3134, y=w3135) -> (x = y?=w3139:bool)
              n1179 = Equal?(x=w3135, y=w3136) -> (x = y?=w3138:bool)
              n1180 = Compound Arithmetic op=AND(w3139, w3138) -> (w3137:bool)
            }
            frame 13 {
              # "A,C e,D ativos"
              n1181 = Equal?(x=w3145, y=w3140) -> (x = y?=w3144:bool)
              n1182 = Equal?(x=w3140, y=w3141) -> (x = y?=w3143:bool)
              n1183 = Compound Arithmetic op=AND(w3144, w3143) -> (w3142:bool)
            }
            frame 12 {
              # "Só C e D ativos"
              n1184 = Equal?(x=w3146, y=w3148) -> (x = y?=w3147:bool)
            }
            frame 11 {
              # "A,B e,D ativos"
              n1185 = Equal?(x=w3154, y=w3153) -> (x = y?=w3152:bool)
              n1186 = Equal?(x=w3153, y=w3149) -> (x = y?=w3151:bool)
              n1187 = Compound Arithmetic op=AND(w3152, w3151) -> (w3150:bool)
            }
            frame 10 {
              # "Só B e D ativos"
              n1188 = Equal?(x=w3155, y=w3157) -> (x = y?=w3156:bool)
            }
            frame 9 {
              # "Só A e D ativos"
              n1189 = Equal?(x=w3160, y=w3159) -> (x = y?=w3158:bool)
            }
            frame 7 {
              # "A,B,C ativos"
              n1190 = Equal?(x=w3166, y=w3165) -> (x = y?=w3163:bool)
              n1191 = Equal?(x=w3165, y=w3164) -> (x = y?=w3162:bool)
              n1192 = Compound Arithmetic op=AND(w3163, w3162) -> (w3161:bool)
            }
            frame 6 {
              # "Só B e C ativos"
              n1193 = Equal?(x=w3169, y=w3168) -> (x = y?=w3167:bool)
            }
            frame 5 {
              # "Só A e C ativos"
              n1194 = Equal?(x=w3172, y=w3171) -> (x = y?=w3170:bool)
            }
            frame 3 {
              # "só A e B ativos"
              n1195 = Equal?(x=w3175, y=w3174) -> (x = y?=w3173:bool)
            }
            frame 0..2, 4, 8, Default {
              # "nenhum ou só 1  \ncanal ativo."
            }
          }
          n1196 = call-dynamic "Write AcquisitionD.vi"("error in (no error)"=w3115, "Acquisition.lvclass"=w3116, "S4ACS_GUI in"=w3114) -> ("error out"=w3105:errorcluster, "S4ACS_GUI out"=w3106:refnum<class "S4GUI.lvclass">)  [unwired: 7 in]
          n1197 = And(x=w3072, y=TRUE) -> (x .and. y?=w3080:bool)
          n1198 = case shown="True" w3080 {
            tunnel: w3106 -> [w3178 w3207]
            tunnel: [w3177 w3206] -> w3065
            tunnel: w3072 -> [w3179 _]
            tunnel: w3066 -> [_ w3205]
            tunnel: w3064 -> [_ w3200]
            frame False {
              n1199 = case shown="True" w3179 {
                tunnel: w3178 -> [w3186 w3199]
                tunnel: [w3190 w3198] -> w3177
                frame False {
                  # "Esperando todos os canais habilitados mudarem de sequesDone.\nE verificando a maior duracao de cubo entre os canais."
                  n1200 = local read "time307"() -> (w3189:u32)
                  n1201 = Tick Count (ms)() -> (millisecond timer value=w3188:u32)
                  n1202 = Subtract(x=w3188, y=w3189) -> (x-y=w3183:u32)
                  n1203 = call-dynamic "GetGreatestCube.vi"("S4GUI in"=w3186) -> ("S4GUI out"=w3185:refnum<class "S4GUI.lvclass">, "greatest (ms)"=w3181:dbl)  [unwired: 8 in, 1 out]
                  n1204 = To Double Precision Float(number=w3183) -> (double precision float=w3187:dbl)
                  n1205 = Add(x=1000.0 ("y"), y=w3181) -> (x+y=w3180:dbl)
                  n1206 = Less?(x=w3180, y=w3187) -> (x < y?=w3184:bool)
                  n1207 = case shown="True" w3184 {
                    tunnel: w3185 -> [w3191 w3195]
                    tunnel: [w3191 w3194] -> w3190
                    frame False {
                    }
                    frame True {
                      n1208 = Bundle By Name(cluster=w3195, "Obs_state"=u32 1, "Error Msg"="ERROR: Acquisition Timeout - HandleObservationSync.vi - state 312.") -> (w3194:refnum<class "S4GUI.lvclass">)
                    }
                  }
                }
                frame True {
                  # "Nunca entra aqui!!"
                  n1209 = Bundle By Name(cluster=w3199, "Obs_state"=u32 1, "Error Msg"="ERROR: Sequence_done not equal in all active channels.") -> (w3198:refnum<class "S4GUI.lvclass">)
                }
              }
            }
            frame True {
              # "STOP?"
              n1210 = local read "time308"() -> (w3203:u32)
              n1211 = Tick Count (ms)() -> (millisecond timer value=w3204:u32)
              n1212 = Subtract(x=w3204, y=w3203) -> (x-y=→"delay Acq":u32)
              n1213 = case shown="False" w3205 {
                tunnel: w3200 -> [_ _]
                tunnel: [u32 303 u32 0] -> w3201
                frame False {
                }
                frame True {
                }
              }
              n1214 = Bundle By Name(cluster=w3207, "Obs_state"=w3201) -> (w3206:refnum<class "S4GUI.lvclass">)
            }
          }
        }
        frame 314 {
          n1215 = Unbundle By Name(w3293) -> ("cyclesDone"=w3291:u32)
          n1216 = Increment(x=w3291) -> (x+1=w3290:u32)
          n1217 = Bundle By Name(cluster=w3293, "cyclesDone"=w3290) -> (w3292:refnum<class "S4GUI.lvclass">)
          n1218 = Unbundle By Name(w3292) -> ("TotalCiclos"=w3300:u32, "cyclesDone"=w3299:u32)
          n1219 = Subtract(x=w3300, y=w3299) -> (x-y=w3298:u32)
          n1220 = Greater Than 0?(x=w3298) -> (x > 0?=w3297:bool)
          n1221 = Select(t=u32 303, s=w3297, f=u32 0) -> (s? t:f=w3296:u32)
          n1222 = Bundle By Name(cluster=w3292, "Obs_state"=w3296) -> (w3301:refnum<class "S4GUI.lvclass">)
        }
        frame 321 {
          n1223 = call-dynamic "Read AcquisitionA.vi"("error in (no error)"=w3365, "S4ACS_GUI in"=w3366) -> ("error out"=w3320:errorcluster, "Acquisition.lvclass"=w3321:refnum<class "Acquisition.lvclass">, "S4ACS_GUI out"=w3368:refnum<class "S4GUI.lvclass">)  [unwired: 7 in]
          n1224 = call-dynamic "Read enabled.vi"("error in (no error)"=w3320, "Server in"=w3321) -> ("error out"=w3319:errorcluster, "enabled"=w3306:bool, "Server out"=w3322:refnum<class "Acquisition.lvclass">)  [unwired: 7 in]
          n1225 = call "Read connection.vi"("error in (no error)"=w3319, "Server in"=w3322) -> ("error out"=w3345:errorcluster, "connection"=w3329:bool, "Server out"=w3346:refnum<class "Acquisition.lvclass">)  [unwired: 7 in]
          n1226 = And(x=w3329, y=w3306) -> (x .and. y?=w3330:bool)
          n1227 = case shown="True" w3330 {
            tunnel: w3346 -> [w3483 w3502]
            tunnel: w3345 -> [w3482 w3501]
            tunnel: [w3483 w3499] -> w3369
            tunnel: [w3482 w3498] -> w3367
            tunnel: [w3479 u32 0 ("New_State")] -> w3335
            tunnel: w3306 -> [w3478 _]
            frame False {
              n1228 = Select(t=u32 1, s=w3478, f=u32 0) -> (s? t:f=w3479:u32)
            }
            frame True {
              n1229 = call-dynamic "Read Channel.vi"("error in (no error)"=w3501, "Acquisition in"=w3502) -> ("error out"=w3485:errorcluster, "Channel.lvclass"=w3488:refnum<class "Channel.lvclass">, "Acquisition out"=w3500:refnum<class "Acquisition.lvclass">)  [unwired: 7 in]
              n1230 = call-dynamic "Write wait_expose.vi"("error in (no error)"=w3485, "wait_expose"=TRUE, "Channel in"=w3488) -> ("error out"=w3484:errorcluster, "Channel out"=w3487:refnum<class "Channel.lvclass">)  [unwired: 7 in]
              n1231 = call-dynamic "Read State Machine.vi"("error in (no error)"=w3484, "Device in"=w3487) -> ("error out"=w3495:errorcluster, "State Machine.lvclass"=w3497:refnum<class "State Machine.lvclass">, "Device out"=w3493:refnum<class "Channel.lvclass">)  [unwired: 7 in]
              n1232 = call "Next State.vi"("error in (no error)"=w3495, "New_State"=40, "State Machine in"=w3497) -> ("error out"=w3490:errorcluster, "State Machine out"=w3491:refnum<class "State Machine.lvclass">)  [unwired: 7 in]
              n1233 = call-dynamic "Write State Machine.vi"("error in (no error)"=w3490, "State Machine.lvclass"=w3491, "Device in"=w3493) -> ("error out"=w3492:errorcluster, "Device out"=w3494:refnum<class "Channel.lvclass">)  [unwired: 7 in]
              n1234 = call-dynamic "Write Channel.vi"("error in (no error)"=w3492, "Channel.lvclass"=w3494, "Acquisition in"=w3500) -> ("error out"=w3498:errorcluster, "Acquisition out"=w3499:refnum<class "Acquisition.lvclass">)  [unwired: 7 in]
            }
          }
          n1235 = call-dynamic "Write AcquisitionA.vi"("error in (no error)"=w3367, "Acquisition.lvclass"=w3369, "S4ACS_GUI in"=w3368) -> ("error out"=w3362:errorcluster, "S4ACS_GUI out"=w3363:refnum<class "S4GUI.lvclass">)  [unwired: 7 in]
          n1236 = call "Read AcquisitionB.vi"("error in (no error)"=w3362, "S4ACS_GUI in"=w3363) -> ("error out"=w3316:errorcluster, "Acquisition.lvclass"=w3318:refnum<class "Acquisition.lvclass">, "S4ACS_GUI out"=w3360:refnum<class "S4GUI.lvclass">)  [unwired: 7 in]
          n1237 = call-dynamic "Read enabled.vi"("error in (no error)"=w3316, "Server in"=w3318) -> ("error out"=w3315:errorcluster, "enabled"=w3305:bool, "Server out"=w3317:refnum<class "Acquisition.lvclass">)  [unwired: 7 in]
          n1238 = call "Read connection.vi"("error in (no error)"=w3315, "Server in"=w3317) -> ("error out"=w3343:errorcluster, "connection"=w3327:bool, "Server out"=w3344:refnum<class "Acquisition.lvclass">)  [unwired: 7 in]
          n1239 = And(x=w3327, y=w3305) -> (x .and. y?=w3328:bool)
          n1240 = case shown="True" w3328 {
            tunnel: w3344 -> [w3458 w3477]
            tunnel: w3343 -> [w3457 w3476]
            tunnel: [w3458 w3474] -> w3361
            tunnel: [w3457 w3473] -> w3359
            tunnel: [w3454 u32 0 ("New_State")] -> w3334
            tunnel: w3305 -> [w3453 _]
            frame False {
              n1241 = Select(t=u32 2, s=w3453, f=u32 0) -> (s? t:f=w3454:u32)
            }
            frame True {
              n1242 = call-dynamic "Read Channel.vi"("error in (no error)"=w3476, "Acquisition in"=w3477) -> ("error out"=w3460:errorcluster, "Channel.lvclass"=w3462:refnum<class "Channel.lvclass">, "Acquisition out"=w3475:refnum<class "Acquisition.lvclass">)  [unwired: 7 in]
              n1243 = call-dynamic "Write wait_expose.vi"("error in (no error)"=w3460, "wait_expose"=TRUE, "Channel in"=w3462) -> ("error out"=w3459:errorcluster, "Channel out"=w3461:refnum<class "Channel.lvclass">)  [unwired: 7 in]
              n1244 = call-dynamic "Read State Machine.vi"("error in (no error)"=w3459, "Device in"=w3461) -> ("error out"=w3470:errorcluster, "State Machine.lvclass"=w3472:refnum<class "State Machine.lvclass">, "Device out"=w3468:refnum<class "Channel.lvclass">)  [unwired: 7 in]
              n1245 = call "Next State.vi"("error in (no error)"=w3470, "New_State"=40, "State Machine in"=w3472) -> ("error out"=w3465:errorcluster, "State Machine out"=w3466:refnum<class "State Machine.lvclass">)  [unwired: 7 in]
              n1246 = call-dynamic "Write State Machine.vi"("error in (no error)"=w3465, "State Machine.lvclass"=w3466, "Device in"=w3468) -> ("error out"=w3467:errorcluster, "Device out"=w3469:refnum<class "Channel.lvclass">)  [unwired: 7 in]
              n1247 = call-dynamic "Write Channel.vi"("error in (no error)"=w3467, "Channel.lvclass"=w3469, "Acquisition in"=w3475) -> ("error out"=w3473:errorcluster, "Acquisition out"=w3474:refnum<class "Acquisition.lvclass">)  [unwired: 7 in]
            }
          }
          n1248 = call "Write AcquisitionB.vi"("error in (no error)"=w3359, "Acquisition.lvclass"=w3361, "S4ACS_GUI in"=w3360) -> ("error out"=w3355:errorcluster, "S4ACS_GUI out"=w3354:refnum<class "S4GUI.lvclass">)  [unwired: 7 in]
          n1249 = call-dynamic "Read AcquisitionC.vi"("error in (no error)"=w3355, "S4ACS_GUI in"=w3354) -> ("error out"=w3312:errorcluster, "Acquisition.lvclass"=w3314:refnum<class "Acquisition.lvclass">, "S4ACS_GUI out"=w3357:refnum<class "S4GUI.lvclass">)  [unwired: 7 in]
          n1250 = call-dynamic "Read enabled.vi"("error in (no error)"=w3312, "Server in"=w3314) -> ("error out"=w3311:errorcluster, "enabled"=w3304:bool, "Server out"=w3313:refnum<class "Acquisition.lvclass">)  [unwired: 7 in]
          n1251 = call "Read connection.vi"("error in (no error)"=w3311, "Server in"=w3313) -> ("error out"=w3341:errorcluster, "connection"=w3324:bool, "Server out"=w3342:refnum<class "Acquisition.lvclass">)  [unwired: 7 in]
          n1252 = And(x=w3324, y=w3304) -> (x .and. y?=w3326:bool)
          n1253 = case shown="True" w3326 {
            tunnel: [w3432 w3446] -> w3358
            tunnel: [w3433 w3445] -> w3356
            tunnel: w3342 -> [w3433 w3443]
            tunnel: w3341 -> [w3432 w3442]
            tunnel: [w3429 u32 0 ("New_State")] -> w3333
            tunnel: w3304 -> [w3428 _]
            frame False {
              n1254 = Select(t=u32 4, s=w3428, f=u32 0) -> (s? t:f=w3429:u32)
            }
            frame True {
              n1255 = call-dynamic "Read Channel.vi"("error in (no error)"=w3442, "Acquisition in"=w3443) -> ("error out"=w3435:errorcluster, "Channel.lvclass"=w3437:refnum<class "Channel.lvclass">, "Acquisition out"=w3444:refnum<class "Acquisition.lvclass">)  [unwired: 7 in]
              n1256 = call-dynamic "Write wait_expose.vi"("error in (no error)"=w3435, "wait_expose"=TRUE, "Channel in"=w3437) -> ("error out"=w3434:errorcluster, "Channel out"=w3436:refnum<class "Channel.lvclass">)  [unwired: 7 in]
              n1257 = call-dynamic "Read State Machine.vi"("error in (no error)"=w3434, "Device in"=w3436) -> ("error out"=w3449:errorcluster, "State Machine.lvclass"=w3447:refnum<class "State Machine.lvclass">, "Device out"=w3451:refnum<class "Channel.lvclass">)  [unwired: 7 in]
              n1258 = call "Next State.vi"("error in (no error)"=w3449, "New_State"=40, "State Machine in"=w3447) -> ("error out"=w3441:errorcluster, "State Machine out"=w3440:refnum<class "State Machine.lvclass">)  [unwired: 7 in]
              n1259 = call-dynamic "Write State Machine.vi"("error in (no error)"=w3441, "State Machine.lvclass"=w3440, "Device in"=w3451) -> ("error out"=w3452:errorcluster, "Device out"=w3450:refnum<class "Channel.lvclass">)  [unwired: 7 in]
              n1260 = call-dynamic "Write Channel.vi"("error in (no error)"=w3452, "Channel.lvclass"=w3450, "Acquisition in"=w3444) -> ("error out"=w3446:errorcluster, "Acquisition out"=w3445:refnum<class "Acquisition.lvclass">)  [unwired: 7 in]
            }
          }
          n1261 = call-dynamic "Write AcquisitionC.vi"("error in (no error)"=w3358, "Acquisition.lvclass"=w3356, "S4ACS_GUI in"=w3357) -> ("error out"=w3352:errorcluster, "S4ACS_GUI out"=w3351:refnum<class "S4GUI.lvclass">)  [unwired: 7 in]
          n1262 = call-dynamic "Read AcquisitionD.vi"("error in (no error)"=w3352, "S4ACS_GUI in"=w3351) -> ("error out"=w3308:errorcluster, "Acquisition.lvclass"=w3310:refnum<class "Acquisition.lvclass">, "S4ACS_GUI out"=w3350:refnum<class "S4GUI.lvclass">)  [unwired: 7 in]
          n1263 = call-dynamic "Read enabled.vi"("error in (no error)"=w3308, "Server in"=w3310) -> ("error out"=w3307:errorcluster, "enabled"=w3303:bool, "Server out"=w3309:refnum<class "Acquisition.lvclass">)  [unwired: 7 in]
          n1264 = call "Read connection.vi"("error in (no error)"=w3307, "Server in"=w3309) -> ("error out"=w3339:errorcluster, "connection"=w3323:bool, "Server out"=w3340:refnum<class "Acquisition.lvclass">)  [unwired: 7 in]
          n1265 = And(x=w3323, y=w3303) -> (x .and. y?=w3325:bool)
          n1266 = case shown="True" w3325 {
            tunnel: w3339 -> [w3407 w3427]
            tunnel: [w3407 w3426] -> w3353
            tunnel: w3340 -> [w3408 w3419]
            tunnel: [w3408 w3417] -> w3349
            tunnel: [w3404 u32 0 ("New_State")] -> w3332
            tunnel: w3303 -> [w3403 _]
            frame False {
              n1267 = Select(t=u32 8, s=w3403, f=u32 0) -> (s? t:f=w3404:u32)
            }
            frame True {
              n1268 = call-dynamic "Read Channel.vi"("error in (no error)"=w3427, "Acquisition in"=w3419) -> ("error out"=w3409:errorcluster, "Channel.lvclass"=w3412:refnum<class "Channel.lvclass">, "Acquisition out"=w3418:refnum<class "Acquisition.lvclass">)  [unwired: 7 in]
              n1269 = call-dynamic "Write wait_expose.vi"("error in (no error)"=w3409, "wait_expose"=TRUE, "Channel in"=w3412) -> ("error out"=w3410:errorcluster, "Channel out"=w3411:refnum<class "Channel.lvclass">)  [unwired: 7 in]
              n1270 = call-dynamic "Read State Machine.vi"("error in (no error)"=w3410, "Device in"=w3411) -> ("error out"=w3423:errorcluster, "State Machine.lvclass"=w3425:refnum<class "State Machine.lvclass">, "Device out"=w3421:refnum<class "Channel.lvclass">)  [unwired: 7 in]
              n1271 = call "Next State.vi"("error in (no error)"=w3423, "New_State"=40, "State Machine in"=w3425) -> ("error out"=w3415:errorcluster, "State Machine out"=w3416:refnum<class "State Machine.lvclass">)  [unwired: 7 in]
              n1272 = call-dynamic "Write State Machine.vi"("error in (no error)"=w3415, "State Machine.lvclass"=w3416, "Device in"=w3421) -> ("error out"=w3420:errorcluster, "Device out"=w3422:refnum<class "Channel.lvclass">)  [unwired: 7 in]
              n1273 = call-dynamic "Write Channel.vi"("error in (no error)"=w3420, "Channel.lvclass"=w3422, "Acquisition in"=w3418) -> ("error out"=w3426:errorcluster, "Acquisition out"=w3417:refnum<class "Acquisition.lvclass">)  [unwired: 7 in]
            }
          }
          n1274 = call-dynamic "Write AcquisitionD.vi"("error in (no error)"=w3353, "Acquisition.lvclass"=w3349, "S4ACS_GUI in"=w3350) -> ("error out"=w3348:errorcluster, "S4ACS_GUI out"=w3347:refnum<class "S4GUI.lvclass">)  [unwired: 7 in]
          n1275 = Compound Arithmetic op=ADD(w3335, w3334, w3333, w3332) -> (w3336:u32)
          n1276 = case shown="0, Default" w3336 {
            tunnel: w3331 -> [w3372 _ _ _ _ _ _ _ _ _ _ _ _ _ _ _]
            tunnel: [w3371 u32 1 ("Obs_state") u32 1 ("Obs_state") u32 1 ("Obs_state") u32 1 ("Obs_state") u32 1 ("Obs_state") u32 1 ("Obs_state") u32 1 ("Obs_state") u32 1 ("Obs_state") u32 1 ("Obs_state") u32 1 ("Obs_state") u32 1 ("Obs_state") u32 1 ("Obs_state") u32 1 ("Obs_state") u32 1 ("Obs_state") u32 1 ("Obs_state")] -> w3337
            tunnel: ["" ("Error Msg") "ERROR: Lost channel 1 connection... - HandleObservationSync.vi state 321" ("Error Msg") "ERROR: Lost channel 2 connection...- HandleObservationSync.vi state 321" ("Error Msg") "ERROR: Lost channels 1 and 2 connection...- HandleObservationSync.vi state 321" ("Error Msg") "ERROR: Lost channel 3 connection...- HandleObservationSync.vi state 321" ("Error Msg") "ERROR: Lost channels 1 and  3 connection...- HandleObservationSync.vi state 321" ("Error Msg") "ERROR:  Lost channels 2 and  3 connection...- HandleObservationSync.vi state 321" ("Error Msg") "ERROR:  Lost channels 1, 2 and  3 connection...- HandleObservationSync.vi state 321" ("Error Msg") "ERROR: Lost channel 4 connection...- HandleObservationSync.vi state 321" ("Error Msg") "ERROR:  Lost channels 1 and 4 connection...- HandleObservationSync.vi state 321" ("Error Msg") "ERROR:  Lost channels 2 and 4 connection...- HandleObservationSync.vi state 321" ("Error Msg") "ERROR: Lost channels 1, 2 and 4 connection...- HandleObservationSync.vi state 321" ("Error Msg") "ERROR: Lost channels 3 and 4 connection...- HandleObservationSync.vi state 321" ("Error Msg") "ERROR: Lost channels 1, 3 and 4 connection...- HandleObservationSync.vi state 321" ("Error Msg") "ERROR: Lost channels 2, 3 and 4 connection...- HandleObservationSync.vi state 321" ("Error Msg") "ERROR: Lost channels 1, 2, 3 and 4 connection...- HandleObservationSync.vi state 321" ("Error Msg")] -> w3338
            frame 0, Default {
              n1277 = Increment(x=w3372) -> (x+1=w3371:u32)
            }
            frame 1 {
            }
            frame 2 {
            }
            frame 3 {
            }
            frame 4 {
            }
            frame 5 {
            }
            frame 6 {
            }
            frame 7 {
            }
            frame 8 {
            }
            frame 9 {
            }
            frame 10 {
            }
            frame 11 {
            }
            frame 12 {
            }
            frame 13 {
            }
            frame 14 {
            }
            frame 15 {
            }
          }
          n1278 = Bundle By Name(cluster=w3347, "Obs_state"=w3337, "Error Msg"=w3338) -> (w3364:refnum<class "S4GUI.lvclass">)
        }
        frame 322 {
